vi "MB_TCP_7024_pp.vi"(6 "N":i32, 9 "timeouts":T1={"conn_timeout"=1000, "reconn_timeout"=3000, "N attempt max"=3, "t_reset_TTL"=120000, "write_timeout"=10, "read_timeout"=500, "period"=100} {"t_reset_TTL" min=10 max=240000 step=1; "period" min=10 max=100000 step=1; "read_timeout" min=10 max=60000 step=1; "write_timeout" min=1 max=60000 step=1; "N attempt max" min=1 max=5 step=1; "reconn_timeout" min=10 max=240000 step=1; "conn_timeout" min=10 max=240000}, 10 "write enable":bool=TRUE, 11 "stop":bool) -> (0 "error out":errorcluster, 2 "errors":u32, 3 "Z3":u32)   [LabVIEW 2019]
uses:
  NI_modbus_upd/NI_modbus_upd.lvlib
  NI_modbus_upd.llb/MB Modbus Command.ctl
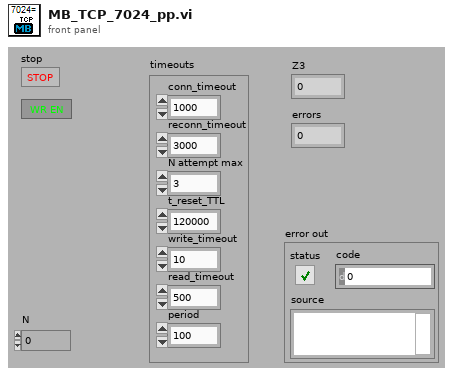
[diagram p1: front panel]
types:
  T1 = cluster{"conn_timeout":i32, "reconn_timeout":u32, "N attempt max":i32, "t_reset_TTL":u32, "write_timeout":i32, "read_timeout":i32, "period":u32}
  T2 = enum16{"Init", "Read", "Read inputs", "Read outputs", "Write", "Write inputs"}
  T3 = enum16{"DI", "DO to write", "DO", "AI", "AO to write", "AO", "DI AI", "DI AO", "DO AI", "DO AO"}
  T4 = enum16{"Start", "Connect", "Write enable", "IP address", "Errors"}
  T5 = typedef "MB Modbus Command.ctl" = cluster{"Function Code":u8, "Starting Address":u16, "Quantity":u16, "Data":u16[], "Discrete":bool[]}
  T6 = cluster{"Transaction ID":u16, "Protocol ID":u16, "Length":u16, "Unit ID":u8}
  T7 = cluster{"Remote IP Address":string, "Remote Port":u16}
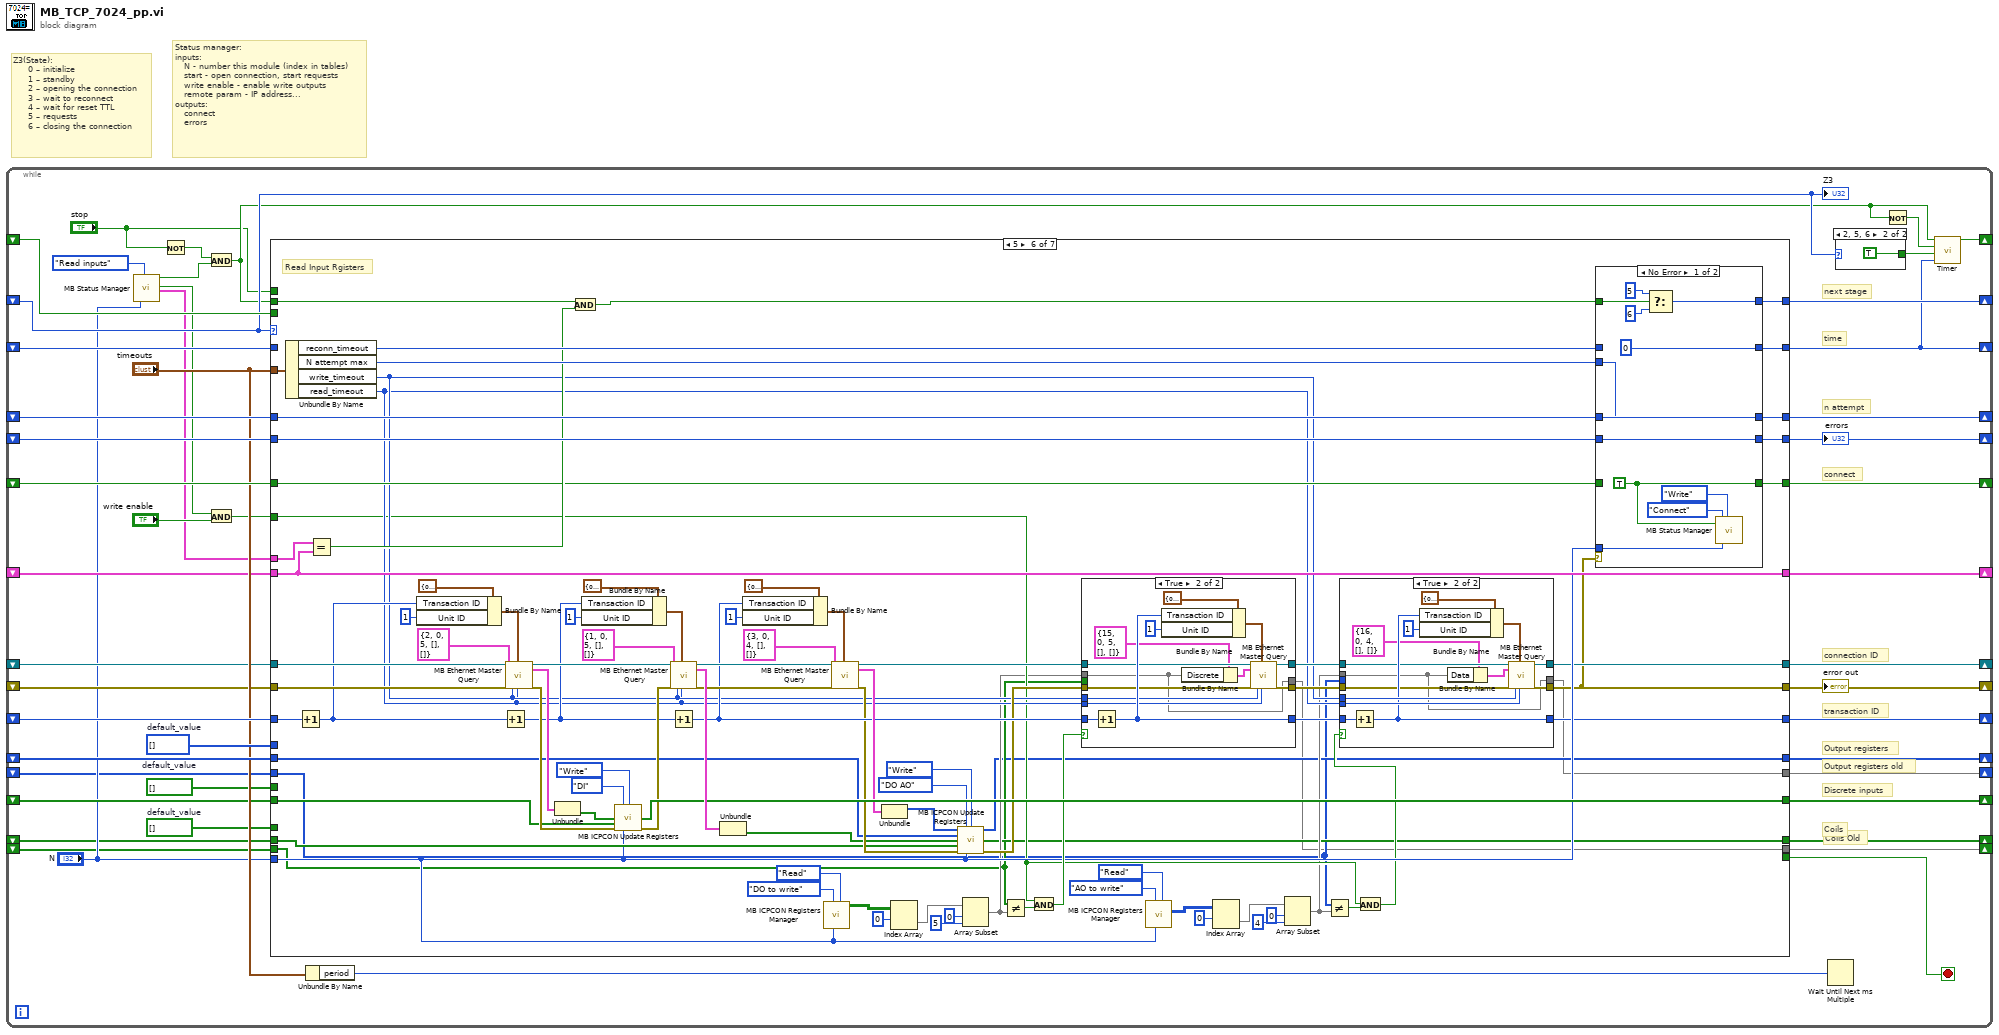
[diagram p0: block diagram]
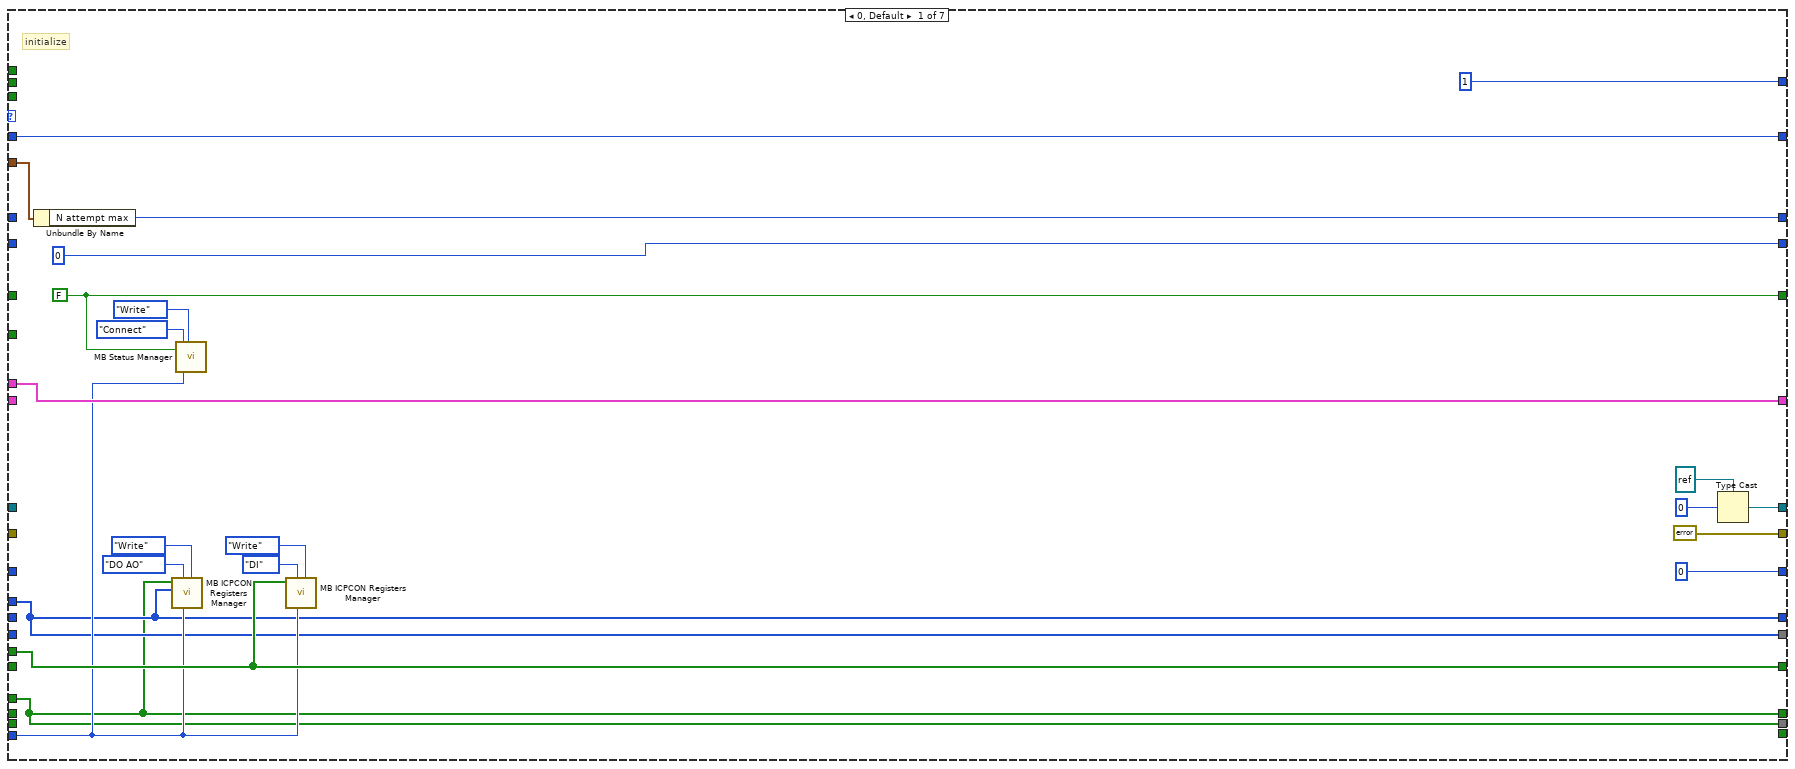
[diagram p2: hidden frame]
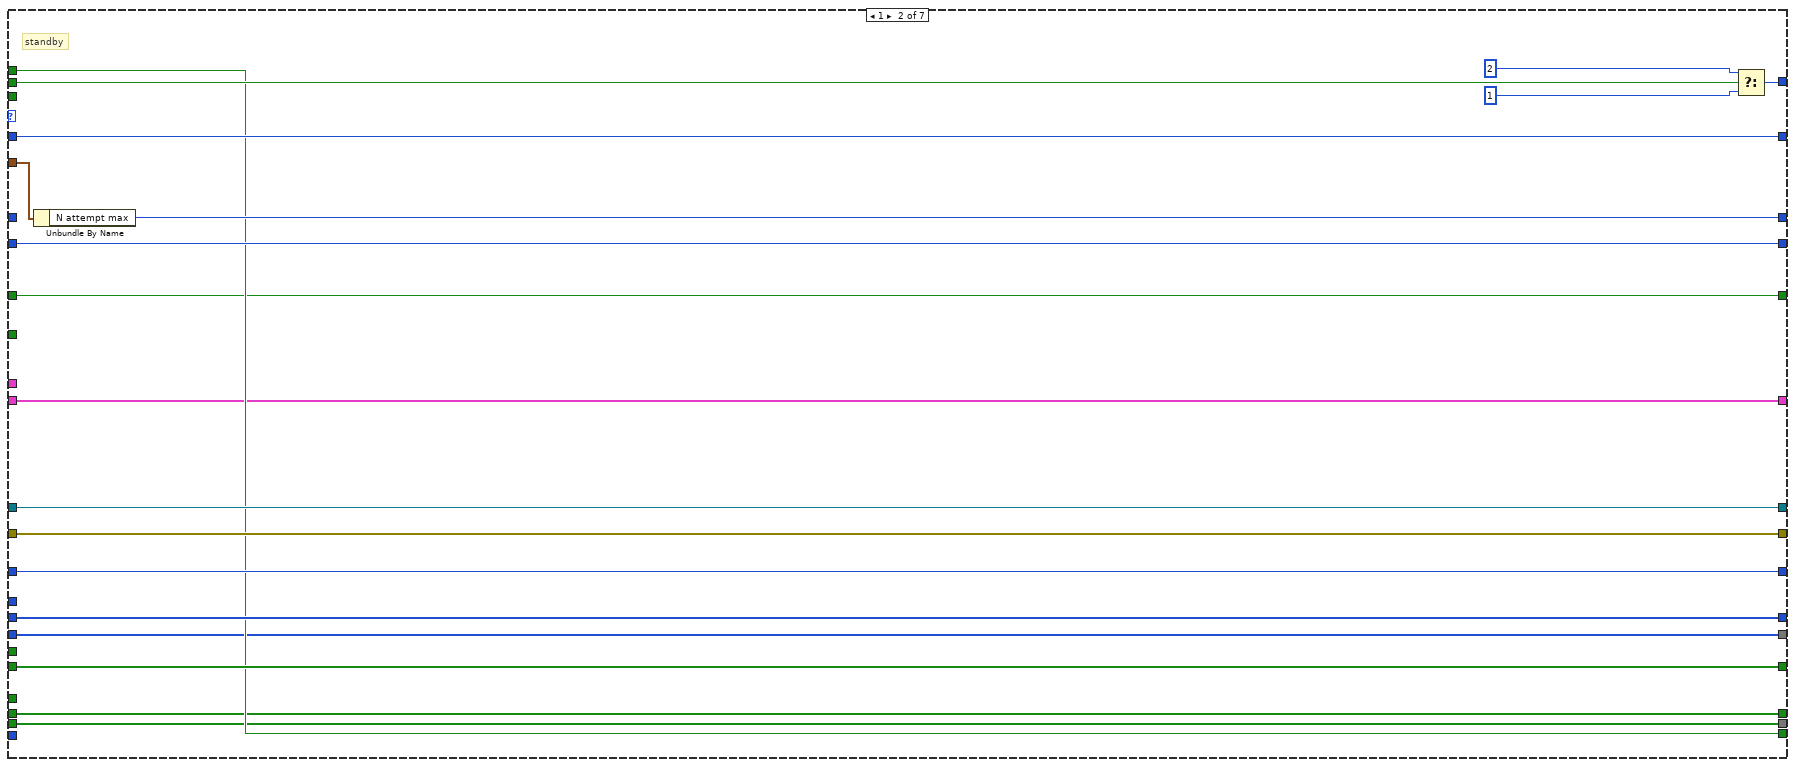
[diagram p3: hidden frame]
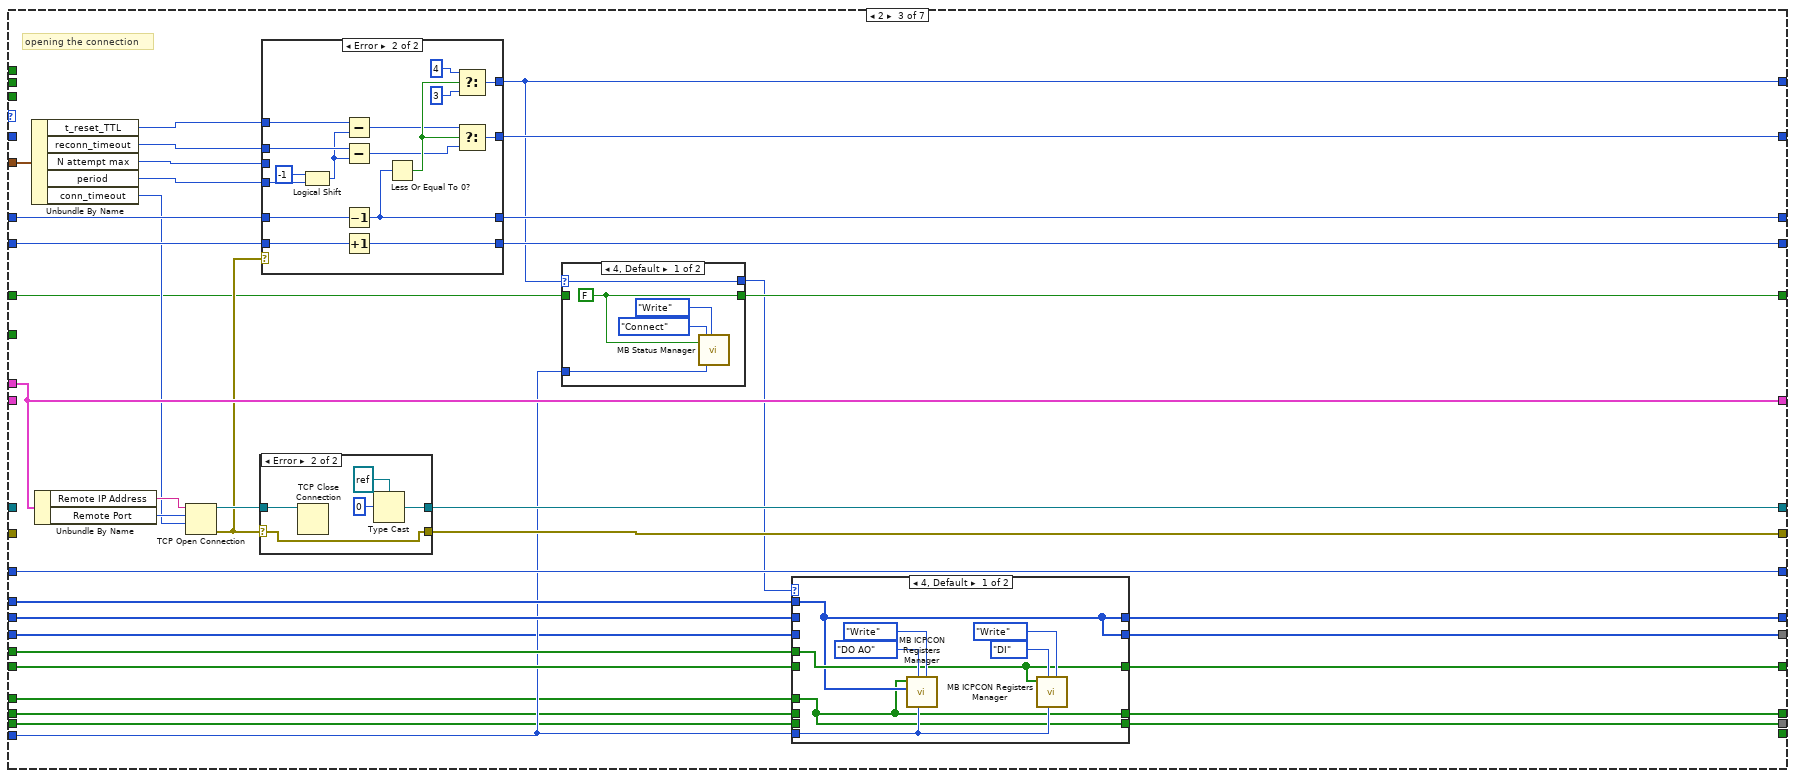
[diagram p4: hidden frame]
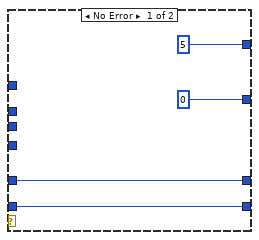
[diagram p8: hidden frame]
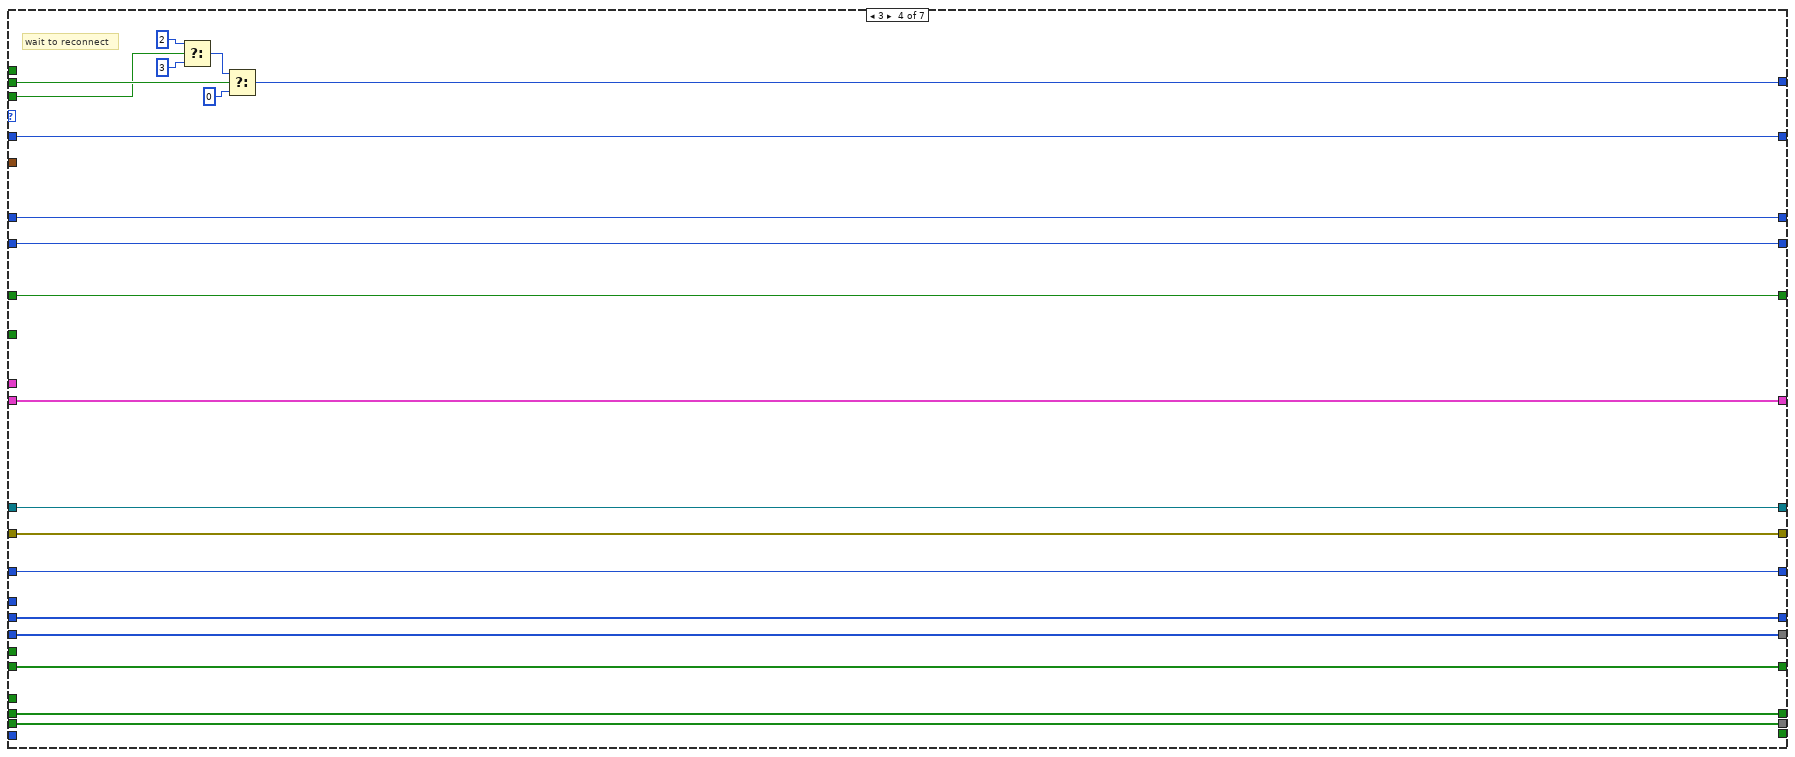
[diagram p9: hidden frame]
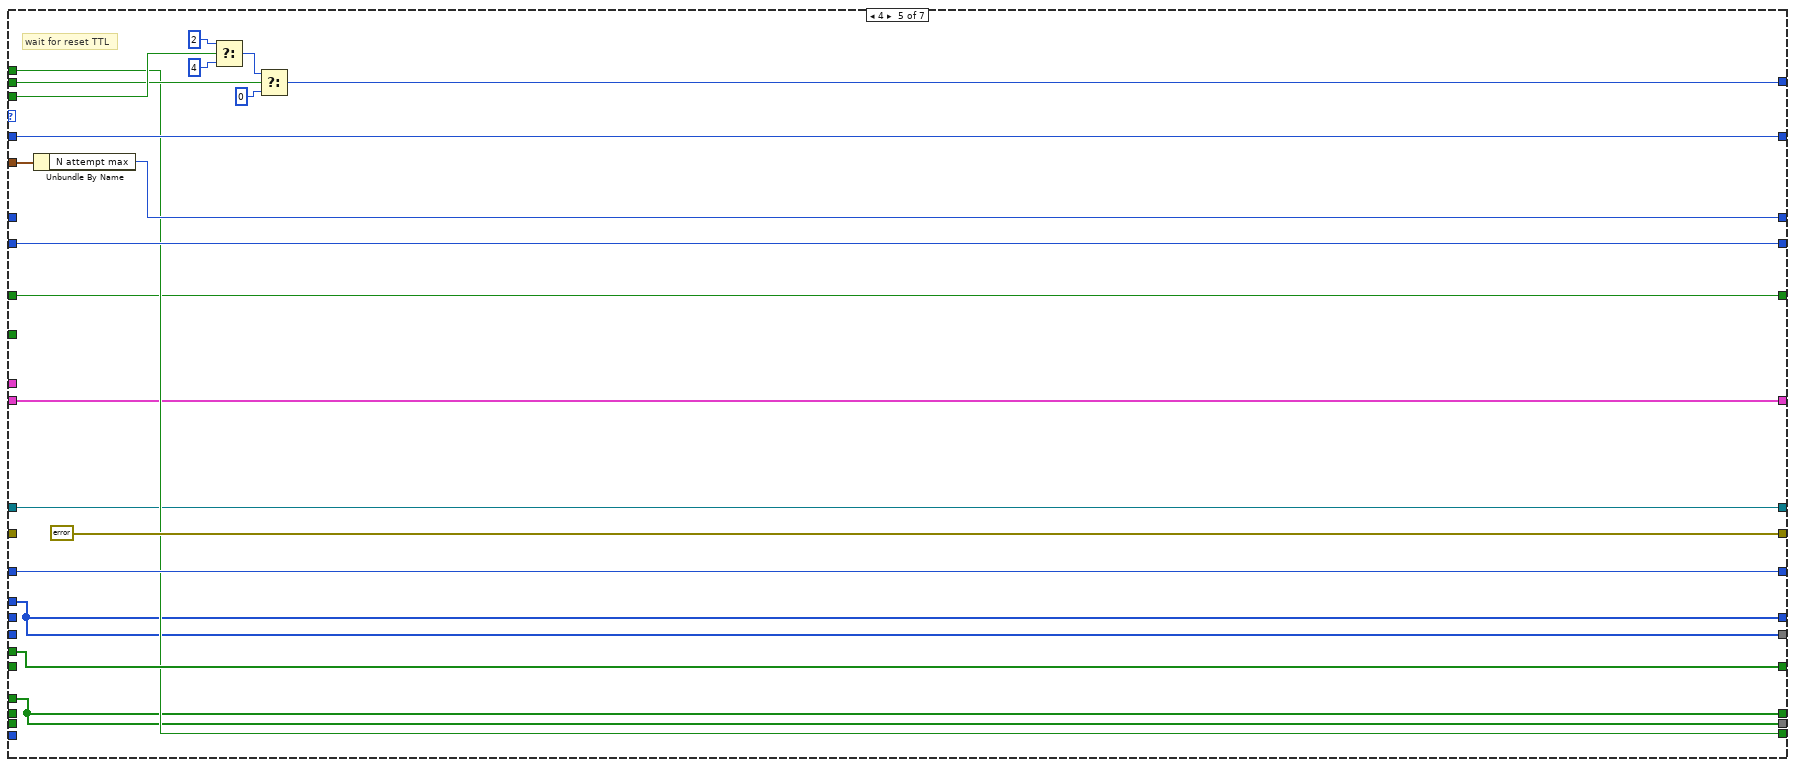
[diagram p10: hidden frame]
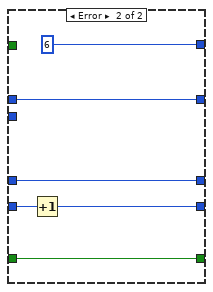
[diagram p13: hidden frame]
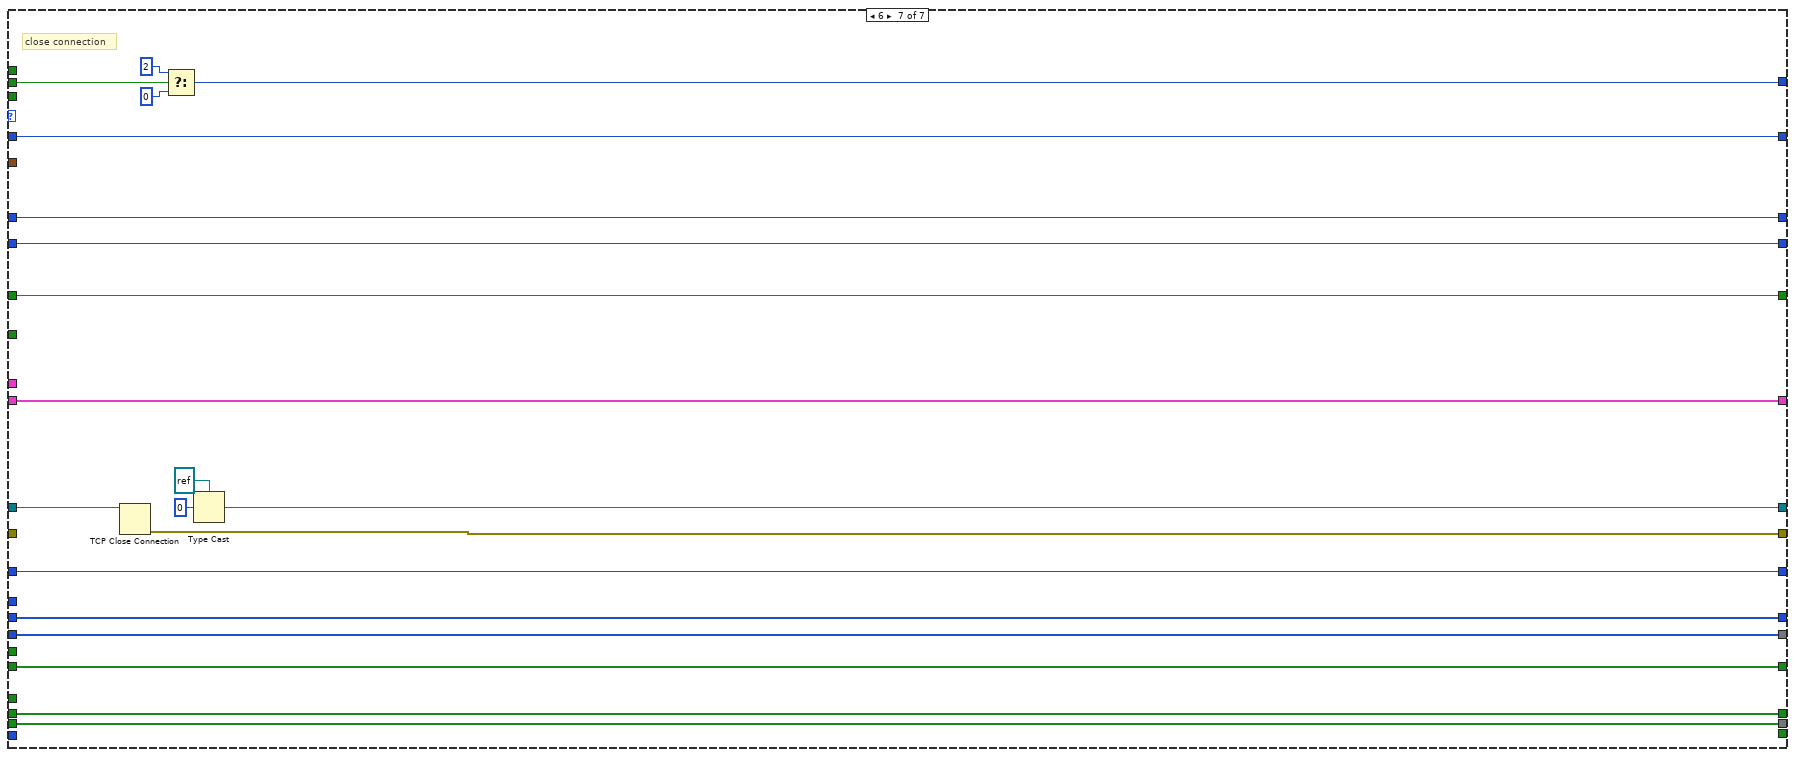
[diagram p14: hidden frame]
diagram:
  # "Status manager:\ninputs:\n   N - number this module (index in tables)\n   start - open connection, start requests\n   write enable - enable write outputs\n   remote param - IP address...\noutputs:\n   connect\n   errors"
  # "Z3(State):\n     0 – initialize \n     1 – standby\n     2 – opening the connection\n     3 – wait to reconnect\n     4 – wait for reset TTL\n     5 – requests\n     6 – closing the connection"
  n1 = while {
    shift-right: [w25] -> _
    shift-left: _ -> [w21]
    shift-right: [w24] -> _
    shift-left: _ -> [w47]
    shift-right: [w46] -> _
    shift-left: _ -> [w44]
    shift-right: [w45] -> _
    shift-left: _ -> [w43]
    shift-right: [w42] -> _
    shift-left: _ -> [w41]
    shift-right: [w40] -> _
    shift-left: _ -> [w26]
    shift-right: [w39] -> _
    shift-left: _ -> [w27]
    shift-right: [w38] -> _
    shift-left: _ -> [w37]
    shift-right: [w36] -> _
    shift-left: _ -> [w35]
    shift-right: [w29] -> _
    shift-left: _ -> [w28]
    shift-right: [w23] -> _
    shift-left: _ -> [w22]
    shift-right: [w14] -> _
    shift-left: _ -> [w13]
    shift-right: [w6] -> _
    shift-left: _ -> [w8]
    shift-right: [w3] -> _
    shift-left: _ -> [w1]
    shift-right: [w4] -> _
    shift-left: _ -> [w2]
    stop <- w17 stop-if-true
    w7 = bool[] []  # default_value
    w30 = bool[] []  # default_value
    w34 = u16[] []  # default_value
    # "Coils Old"
    # "Output registers old"
    # "Coils"
    # "Discrete inputs"
    # "Output registers"
    # "connect"
    # "connection ID"
    # "transaction ID"
    # "n attempt"
    # "time"
    # "next stage"
    n2 = call "MB Status Manager.vi"("N"="N", "Function"=T2."Read inputs") -> ("start"=w12:bool, "write enable"=w11:bool, "Remote Param"=w10:T7)  [unwired: 12 in, 3 out]
    n3 = Not(x="stop") -> (.not. x?=w19:bool)
    n4 = And(x=w19, y=w12) -> (x .and. y?=w20:bool)
    n5 = And(x=w11, y="write enable") -> (x .and. y?=w16:bool)
    n6 = case shown="5" w21 {
      tunnel: [w68 w80 w104 w191 w198 w231 w375] -> w40
      tunnel: [errorcluster {"status"=FALSE, "code"=0, "source"=""} ("error out") w79 w102 w190 errorcluster {"status"=FALSE, "code"=0, "source"=""} ("error out") w229 w376] -> w39
      tunnel: w26 -> [_ w80 _ w191 w198 w295 w372]
      tunnel: w27 -> [_ w79 _ w190 _ w294 _]
      tunnel: [w57 w75 w100 w179 w197 w282 w363] -> w42
      tunnel: w41 -> [_ w75 w101 w179 w197 w283 w363]
      tunnel: w10 -> [w60 _ w107 _ _ w289 _]
      tunnel: [w50 w81 w112 w178 w195 w217 w362] -> w36
      tunnel: w35 -> [_ w81 w113 w178 _ w243 w362]
      tunnel: w37 -> [_ w89 w126 w193 w213 w304 w377]
      tunnel: [u16 0 ("x") w89 w126 w193 w213 w227 w377] -> w38
      tunnel: [w62 w85 w121 w192 w209 w302 w369] -> w46
      tunnel: w44 -> [_ _ w122 w192 _ w302 w369]
      tunnel: [u32 0 ("N attempt max") w88 w124 w189 w212 w301 w374] -> w45
      tunnel: w43 -> [_ w88 w125 w189 w212 w300 w374]
      tunnel: [w64 w87 w118 w188 w211 w297 w373] -> w24
      tunnel: w47 -> [w64 w87 _ w188 w211 _ w373]
      tunnel: "timeouts" -> [w63 w86 w123 _ w210 w303 _]
      tunnel: w20 -> [_ w77 _ w184 w200 w288 w370]
      tunnel: [u32 1 w82 w98 w180 w204 w296 w364] -> w25
      tunnel: w22 -> [_ _ _ w182 w203 _ _]
      tunnel: w34 -> [w50 _ w111 _ w195 _ _]
      tunnel: w30 -> [w53 _ w108 _ w201 _ _]
      tunnel: [w53 w78 w109 w181 w201 w272 w367] -> w29
      tunnel: w28 -> [_ w78 w110 w181 _ w245 w367]
      tunnel: "N" -> [w52 _ w99 _ _ w234 _]
      tunnel: "stop" -> [_ w76 _ _ w199 _ _]
      tunnel: [_ w76 _ _ w199 _ _] -> w17
      tunnel: w16 -> [_ _ _ _ _ w223 _]
      tunnel: [w60 w74 w107 w177 w196 w286 w361] -> w14
      tunnel: w13 -> [_ w74 _ w177 w196 w286 w361]
      tunnel: w7 -> [w49 _ w96 _ w194 _ _]
      tunnel: w8 -> [_ w73 w95 w176 _ w241 w360]
      tunnel: [w49 w73 w94 w176 w194 w219 w360] -> w6
      tunnel: [w50 w72 w91 w175 w195 w215 w359] -> w4
      tunnel: [w49 w71 w90 w174 w194 w214 w358] -> w3
      tunnel: w2 -> [_ w72 w93 w175 _ w216 w359]
      tunnel: w1 -> [_ w71 w92 w174 _ w218 w358]
      frame 0, Default {
        w57 = FALSE ("connect")
        # "initialize"
        n7 = Unbundle By Name(w63) -> ("N attempt max"=w62:i32)
        n8 = call "MB ICPCON Registers Manager.vi"("Function"=enum16{"Init", "Read", "Write", "Read All"}."Write", "N"=w52, "Table"=T3."DO AO", "Registers In"=w50, "Discrete in"=w49) -> ()  [unwired: 4 in, 3 out]
        n9 = call "MB Status Manager.vi"("connect in"=w57, "Table"=T4."Connect", "N"=w52, "Function"=T2."Write") -> ()  [unwired: 10 in, 6 out]
        n10 = call "MB ICPCON Registers Manager.vi"("Function"=enum16{"Init", "Read", "Write", "Read All"}."Write", "N"=w52, "Table"=T3."DI", "Discrete in"=w53) -> ()  [unwired: 5 in, 3 out]
        n11 = Type Cast(type=refnum<k5> refnum ("connection ID"), x=u32 0) -> (*(type *) &x=w68:refnum<k5>)
      }
      frame 1 {
        # "standby"
        n12 = Unbundle By Name(w86) -> ("N attempt max"=w85:i32)
        n13 = Select(t=u32 2, s=w77, f=u32 1) -> (s? t:f=w82:u32)
      }
      frame 2 {
        # "opening the connection"
        n14 = Unbundle By Name(w123) -> ("t_reset_TTL"=w117:u32, "reconn_timeout"=w119:u32, "N attempt max"=w120:i32, "period"=w114:u32, "conn_timeout"=w106:i32)
        n15 = Unbundle By Name(w107) -> ("Remote IP Address"=w116:string, "Remote Port"=w115:u16)
        n16 = TCP Open Connection(address=w116, remote port or service name=w115, timeout ms (60000)=w106) -> (connection ID=w105:refnum<k5>, error out=w103:errorcluster)  [unwired: 2 in]
        n17 = case shown="Error" w103 {
          selector: w103 -> [w134 w136]
          tunnel: w105 -> [w135 w139]
          tunnel: [w135 w138] -> w104
          tunnel: [w134 w136] -> w102
          frame No Error {
          }
          frame Error {
            n18 = TCP Close Connection(connection ID=w139) -> ()  [unwired: 2 in, 2 out]
            n19 = Type Cast(type=refnum<k5> refnum ("connection ID"), x=u32 0) -> (*(type *) &x=w138:refnum<k5>)
          }
        }
        n20 = case shown="Error" w103 {
          tunnel: w125 -> [w157 w173]
          tunnel: [w157 w172] -> w124
          tunnel: w122 -> [w156 w171]
          tunnel: [w156 w170] -> w121
          tunnel: w120 -> [_ _]
          tunnel: [u32 5 w167] -> w98
          tunnel: w119 -> [_ w166]
          tunnel: [u32 0 w165] -> w118
          tunnel: w117 -> [_ w162]
          tunnel: w114 -> [_ w160]
          frame No Error {
          }
          frame Error {
            n21 = Logical Shift(y=i16 -1, x=w160) -> (x << y=w158:u32)
            n22 = Subtract(x=w162, y=w158) -> (x-y=w161:u32)
            n23 = Subtract(x=w166, y=w158) -> (x-y=w163:u32)
            n24 = Decrement(x=w171) -> (x-1=w170:i32)
            n25 = Increment(x=w173) -> (x+1=w172:u32)
            n26 = Less Or Equal To 0?(x=w170) -> (x <= 0?=w164:bool)
            n27 = Select(t=u32 4, s=w164, f=u32 3) -> (s? t:f=w167:u32)
            n28 = Select(t=w161, s=w164, f=w163) -> (s? t:f=w165:u32)
          }
        }
        n29 = case shown="4, Default" w98 {
          selector: w98 -> [w128 w132]
          tunnel: w99 -> [w129 _]
          tunnel: [w130 w133] -> w100
          tunnel: w101 -> [_ w133]
          tunnel: [w128 w132] -> w97
          frame 4, Default {
            w130 = FALSE ("f")
            n30 = call "MB Status Manager.vi"("connect in"=w130, "Table"=T4."Connect", "N"=w129, "Function"=T2."Write") -> ()  [unwired: 10 in, 6 out]
          }
          frame 3, 5 {
          }
        }
        n31 = case shown="4, Default" w97 {
          tunnel: w99 -> [w144 _]
          tunnel: [w142 w153] -> w112
          tunnel: w113 -> [_ w153]
          tunnel: w111 -> [w142 _]
          tunnel: w110 -> [_ w152]
          tunnel: [w143 w152] -> w109
          tunnel: w108 -> [w143 _]
          tunnel: w96 -> [w141 _]
          tunnel: [w141 w151] -> w94
          tunnel: w95 -> [_ w151]
          tunnel: w93 -> [_ w150]
          tunnel: [w142 w150] -> w91
          tunnel: w92 -> [_ w149]
          tunnel: [w141 w149] -> w90
          frame 4, Default {
            n32 = call "MB ICPCON Registers Manager.vi"("Function"=enum16{"Init", "Read", "Write", "Read All"}."Write", "N"=w144, "Table"=T3."DO AO", "Registers In"=w142, "Discrete in"=w141) -> ()  [unwired: 4 in, 3 out]
            n33 = call "MB ICPCON Registers Manager.vi"("Function"=enum16{"Init", "Read", "Write", "Read All"}."Write", "N"=w144, "Table"=T3."DI", "Discrete in"=w143) -> ()  [unwired: 5 in, 3 out]
          }
          frame 3, 5 {
          }
        }
      }
      frame 3 {
        # "wait to reconnect"
        n34 = Select(t=u32 2, s=w182, f=u32 3) -> (s? t:f=w183:u32)
        n35 = Select(t=w183, s=w184, f=u32 0) -> (s? t:f=w180:u32)
      }
      frame 4 {
        # "wait for reset TTL"
        n36 = Unbundle By Name(w210) -> ("N attempt max"=w209:i32)
        n37 = Select(t=u32 2, s=w203, f=u32 4) -> (s? t:f=w205:u32)
        n38 = Select(t=w205, s=w200, f=u32 0) -> (s? t:f=w204:u32)
      }
      frame 5 {
        # "Read Input Rgisters"
        n39 = Unbundle By Name(w303) -> ("reconn_timeout"=w298:u32, "N attempt max"=w299:i32, "write_timeout"=w226:i32, "read_timeout"=w225:i32)
        n40 = Increment(x=w304) -> (x+1=w276:u16)
        n41 = Equal?(x=w289, y=w286) -> (x = y?=w285:bool)
        n42 = Bundle By Name(cluster=T6 {"Transaction ID"=0, "Protocol ID"=0, "Length"=0, "Unit ID"=0} ("MBAP Header"), "Transaction ID"=w276, "Unit ID"=u8 1) -> (w290:T6)
        n43 = Increment(x=w276) -> (x+1=w260:u16)
        n44 = call "MB Ethernet Master Query.vi"("TCP Connection Refnum in"=w295, "Modbus Command"=T5 {"Function Code"=2, "Starting Address"=0, "Quantity"=5, "Data"=[], "Discrete"=[]}, "error in (no error)"=w294, "Write Timeout"=w226, "MBAP Header"=w290, "Read Timeout"=w225) -> ("TCP Connection Refnum (dup)"=w270:refnum<k5>, "Registers"=w293:cluster{"Registers":u16[], "Discrete":bool[]}, "error out"=w269:errorcluster)  [unwired: 9 in, 2 out]
        n45 = Unbundle(w293) -> ("Discrete"=w246:bool[])  [unwired: 1 out]
        n46 = And(x=w288, y=w285) -> (x .and. y?=w287:bool)
        n47 = Bundle By Name(cluster=T6 {"Transaction ID"=0, "Protocol ID"=0, "Length"=0, "Unit ID"=0} ("MBAP Header"), "Transaction ID"=w260, "Unit ID"=u8 1) -> (w279:T6)
        n48 = call "MB ICPCON Update Registers.vi"("Table"=T3."DI", "Function"=enum16{"Init", "Read", "Write", "Read All"}."Write", "Discrete in"=w246, "Default Discrete in"=w245, "error in (no error)"=w269, "N"=w234) -> ("Discretes"=w272:bool[], "error out"=w268:errorcluster)  [unwired: 7 in, 1 out]
        n49 = call "MB Ethernet Master Query.vi"("TCP Connection Refnum in"=w270, "Modbus Command"=T5 {"Function Code"=1, "Starting Address"=0, "Quantity"=5, "Data"=[], "Discrete"=[]} ("MODBUS Command"), "error in (no error)"=w268, "Write Timeout"=w226, "MBAP Header"=w279, "Read Timeout"=w225) -> ("TCP Connection Refnum (dup)"=w262:refnum<k5>, "Registers"=w274:cluster{"Registers":u16[], "Discrete":bool[]}, "error out"=w259:errorcluster)  [unwired: 9 in, 2 out]
        n50 = Increment(x=w260) -> (x+1=w258:u16)
        n51 = Unbundle(w274) -> ("Discrete"=w242:bool[])  [unwired: 1 out]
        n52 = Bundle By Name(cluster=T6 {"Transaction ID"=0, "Protocol ID"=0, "Length"=0, "Unit ID"=0} ("MBAP Header"), "Transaction ID"=w258, "Unit ID"=u8 1) -> (w263:T6)
        n53 = call "MB ICPCON Registers Manager.vi"("Function"=enum16{"Init", "Read", "Write", "Read All"}."Read", "N"=w234, "Table"=T3."DO to write") -> ("Discretes"=w253:bool[][])  [unwired: 6 in, 2 out]
        n54 = call "MB Ethernet Master Query.vi"("TCP Connection Refnum in"=w262, "Modbus Command"=T5 {"Function Code"=3, "Starting Address"=0, "Quantity"=4, "Data"=[], "Discrete"=[]} ("MODBUS Command"), "error in (no error)"=w259, "MBAP Header"=w263) -> ("TCP Connection Refnum (dup)"=w261:refnum<k5>, "Registers"=w267:cluster{"Registers":u16[], "Discrete":bool[]}, "error out"=w248:errorcluster)  [unwired: 11 in, 2 out]
        n55 = Unbundle(w267) -> ("Registers"=w244:u16[])  [unwired: 1 out]
        n56 = Index Array(array=w253, index (row)=0) -> (element=w251:bool[])  [unwired: 1 in]
        n57 = call "MB ICPCON Update Registers.vi"("Registers In"=w244, "Table"=T3."DO AO", "Function"=enum16{"Init", "Read", "Write", "Read All"}."Write", "Default Registers In"=w243, "Discrete in"=w242, "Default Discrete in"=w241, "error in (no error)"=w248, "N"=w234) -> ("Registers"=w217:u16[], "Discretes"=w219:bool[], "error out"=w247:errorcluster)  [unwired: 5 in]
        n58 = Array Subset(array=w251, index=0, length=5) -> (w221:bool[])
        n59 = Not Equal?(x=w218, y=w221) -> (x != y?=w273:bool)
        n60 = And(x=w223, y=w273) -> (x .and. y?=w271:bool)
        n61 = case shown="True" w271 {
          tunnel: w225 -> [_ w331]
          tunnel: w226 -> [_ w330]
          tunnel: w258 -> [w325 w338]
          tunnel: [w325 w337] -> w228
          tunnel: w247 -> [w324 w335]
          tunnel: [w324 w334] -> w230
          tunnel: w261 -> [w326 w333]
          tunnel: [w326 w332] -> w232
          tunnel: w221 -> [_ w327]
          tunnel: w218 -> [w323 _]
          tunnel: [w323 w327] -> w214
          frame False {
          }
          frame True {
            n62 = Increment(x=w338) -> (x+1=w337:u16)
            n63 = Bundle By Name(cluster=T6 {"Transaction ID"=0, "Protocol ID"=0, "Length"=0, "Unit ID"=0} ("MBAP Header"), "Transaction ID"=w337, "Unit ID"=u8 1) -> (w339:T6)
            n64 = Bundle By Name(cluster=T5 {"Function Code"=15, "Starting Address"=0, "Quantity"=5, "Data"=[], "Discrete"=[]} ("MODBUS Command"), "Discrete"=w327) -> (w328:T5)
            n65 = call "MB Ethernet Master Query.vi"("TCP Connection Refnum in"=w333, "Modbus Command"=w328, "error in (no error)"=w335, "Write Timeout"=w330, "MBAP Header"=w339, "Read Timeout"=w331) -> ("TCP Connection Refnum (dup)"=w332:refnum<k5>, "error out"=w334:errorcluster)  [unwired: 9 in, 3 out]
          }
        }
        n66 = call "MB ICPCON Registers Manager.vi"("Function"=enum16{"Init", "Read", "Write", "Read All"}."Read", "N"=w234, "Table"=T3."AO to write") -> ("Registers"=w233:u16[][])  [unwired: 6 in, 2 out]
        n67 = Index Array(array=w233, index (row)=0) -> (element=w240:u16[])  [unwired: 1 in]
        n68 = Array Subset(array=w240, index=0, length=4) -> (w220:u16[])
        n69 = Not Equal?(x=w216, y=w220) -> (x != y?=w224:bool)
        n70 = And(x=w223, y=w224) -> (x .and. y?=w222:bool)
        n71 = case shown="True" w222 {
          tunnel: w225 -> [_ w320]
          tunnel: w226 -> [_ w319]
          tunnel: w228 -> [w307 w318]
          tunnel: [w307 w317] -> w227
          tunnel: w230 -> [w306 w315]
          tunnel: [w306 w314] -> w229
          tunnel: w232 -> [w308 w313]
          tunnel: [w308 w312] -> w231
          tunnel: w220 -> [_ w309]
          tunnel: w216 -> [w305 _]
          tunnel: [w305 w309] -> w215
          frame False {
          }
          frame True {
            n72 = Increment(x=w318) -> (x+1=w317:u16)
            n73 = Bundle By Name(cluster=T6 {"Transaction ID"=0, "Protocol ID"=0, "Length"=0, "Unit ID"=0} ("MBAP Header"), "Transaction ID"=w317, "Unit ID"=u8 1) -> (w321:T6)
            n74 = Bundle By Name(cluster=T5 {"Function Code"=16, "Starting Address"=0, "Quantity"=4, "Data"=[], "Discrete"=[]} ("MODBUS Command"), "Data"=w309) -> (w310:T5)
            n75 = call "MB Ethernet Master Query.vi"("TCP Connection Refnum in"=w313, "Modbus Command"=w310, "error in (no error)"=w315, "Write Timeout"=w319, "MBAP Header"=w321, "Read Timeout"=w320) -> ("TCP Connection Refnum (dup)"=w312:refnum<k5>, "error out"=w314:errorcluster)  [unwired: 9 in, 3 out]
          }
        }
        n76 = case shown="No Error" w229 {
          tunnel: w300 -> [w345 w357]
          tunnel: [w345 w356] -> w301
          tunnel: [w347 u32 6] -> w296
          tunnel: w302 -> [_ w354]
          tunnel: w299 -> [w351 _]
          tunnel: [w351 w354] -> _
          tunnel: w298 -> [_ w353]
          tunnel: [u32 0 w353] -> w297
          tunnel: w287 -> [w346 _]
          tunnel: w283 -> [_ w352]
          tunnel: [w343 w352] -> w282
          tunnel: w234 -> [w342 _]
          frame No Error {
            w343 = TRUE ("f")
            n77 = Select(t=u32 5, s=w346, f=u32 6) -> (s? t:f=w347:u32)
            n78 = call "MB Status Manager.vi"("connect in"=w343, "Table"=T4."Connect", "N"=w342, "Function"=T2."Write") -> ()  [unwired: 10 in, 6 out]
          }
          frame Error {
            n79 = Increment(x=w357) -> (x+1=w356:u32)
          }
        }
      }
      frame 6 {
        # "close connection"
        n80 = TCP Close Connection(connection ID=w372) -> (error out=w376:errorcluster)  [unwired: 2 in, 1 out]
        n81 = Select(t=u32 2, s=w370, f=u32 0) -> (s? t:f=w364:u32)
        n82 = Type Cast(type=refnum<k5> refnum ("connection ID"), x=u32 0) -> (*(type *) &x=w375:refnum<k5>)
      }
    }
    "error out" <- w39
    "errors" <- w45
    n83 = Unbundle By Name("timeouts") -> ("period"=w32:u32)
    n84 = Wait Until Next ms Multiple(millisecond multiple=w32) -> ()  [unwired: 1 out]
    n85 = case shown="2, 5, 6" w21 {
      tunnel: [_ TRUE] -> w31
      frame 0, Default {
      }
      frame 2, 5, 6 {
      }
    }
    n86 = Not(x=w20) -> (.not. x?=w48:bool)
    n87 = call "Timer.vi"("ms"=w24, "Load (F)"=w31, "Reset (F)"=w48, "Start (T)"=w20) -> ("End"=w23:bool)  [unwired: 5 in, 1 out]
    "Z3" <- w21
  }
